vi "homework3.vi"() -> ()   [LabVIEW 2017]
uses:
  <vilib>/Utility/file.llb/Write Delimited Spreadsheet (DBL).vi
panel:
  in  "操作(0:open)":T1(ring)
  in  "名称或相对路径":string
  out "数组":dbl[][](array[numeric])
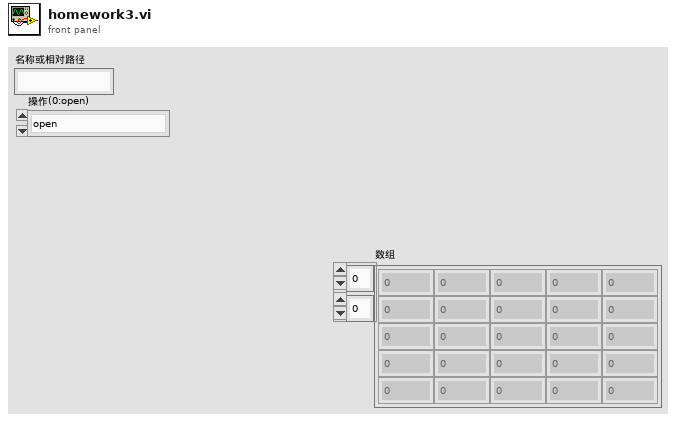
[diagram p1: front panel]
types:
  T1 = enum16{"open", "replace", "create", "open or create", "replace or create", "replace or create with confirmation"}
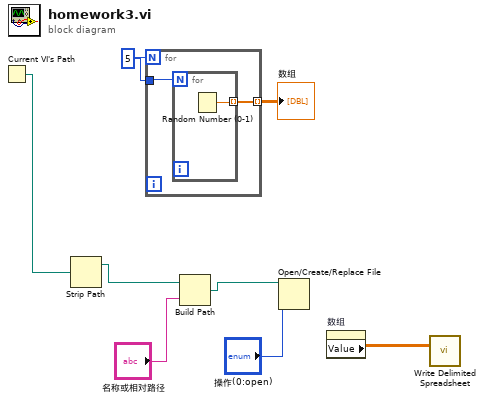
[diagram p0: block diagram]
diagram:
  w8 = 5
  n1 = Current VI's Path() -> (path=w6:path)
  n2 = Strip Path(path=w6) -> (stripped path=w5:path)  [unwired: 1 out]
  n3 = for {
    N: w8 -> [_]
    tunnel: w8 -> [w10]
    tunnel: [w9] -> w7 mode=indexing
    n4 = for {
      N: w10 -> [_]
      tunnel: [w11] -> w9 mode=indexing
      n5 = Random Number (0-1)() -> (number: 0 to 1=w11:dbl)
    }
  }
  "数组" <- w7
  n6 = Build Path(base path=w5, name or relative path="名称或相对路径") -> (appended path=w3:path)
  n7 = Open/Create/Replace File(file path (use dialog)=w3, operation (0:open)="操作(0:open)") -> ()  [unwired: 4 in, 3 out]
  n8 = property on="数组" class="Arr (严格)"() -> ("Value"=w1:dbl[][])  [unwired: 2 in, 2 out]
  n9 = call-poly <vilib>:"Write Delimited Spreadsheet.vi"("2D data"=w1) -> ()  [unwired: 13 in, 2 out]
